vi "Set Lamp intensity.vi"(8 "error in (no error)":errorcluster {"code" format="%.0x"}, 9 "Lamp Intensity (1.0 V)":dbl=1.0, 10 "Device Number (1)":i32=1, 11 "VISA Resource Name":refnum<visa-resource-name>) -> (0 "error out":errorcluster {"code" format="%.0x"}, 3 "VISA Resource Name Out":refnum<visa-resource-name>)   [LabVIEW 2018, in "Olympus IX BX Series.lvlib"]
doc: "Sets the voltage of the lamp for transmitted light / reflected light."
uses:
  Olympus IX BX Series.lvlib
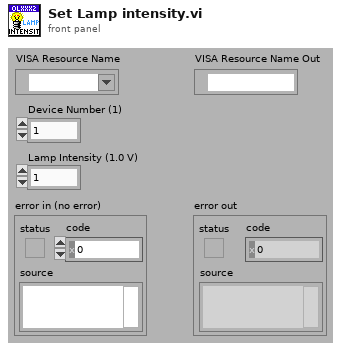
[diagram p1: front panel]
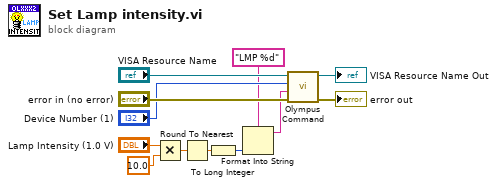
[diagram p0: block diagram]
diagram:
  n1 = Multiply(x="Lamp Intensity (1.0 V)", y=10.0) -> (x*y=w5:dbl)
  n2 = Round To Nearest(number=w5) -> (nearest integer value=w4:dbl)
  n3 = To Long Integer(number=w4) -> (32bit integer=w3:i32)
  n4 = Format Into String(format string="LMP %d", w3) -> (resulting string=w2:string)  [unwired: 2 in, 1 out]
  n5 = call "Olympus Command.vi"("error in (no error)"="error in (no error)", "Command string"=w2, "Device Number (1)"="Device Number (1)", "VISA Resource Name"="VISA Resource Name") -> ("error out"=→"error out":errorcluster, "VISA Resource Name Out"=→"VISA Resource Name Out":refnum<visa-resource-name>)  [unwired: 5 in, 1 out]
